vi "CODMn启动 (子VI).vi"(9 "强制切换":bool, 10 "CODMn量程切换":enum32{"H", "L", "AUTO"}(ring)=enum."AUTO", 11 "启动测量模式":T2) -> (0 "error out":T1={"status"=FALSE, "代码"=4, "source"=""} caption="错误输出" {"代码" items=["执行成功"=1, "执行失败，但不知道原因"=2, "命令请求条件错误"=3, "通讯超时"=4, "系统繁忙不能执行"=5, "系统故障"=6, "没有数据"=100]})   [LabVIEW 2016]
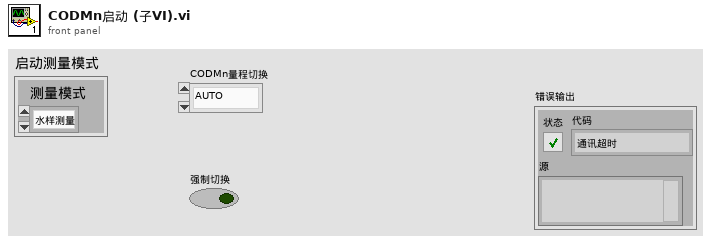
[diagram p1: front panel]
types:
  T1 = cluster{"status":bool, "代码":u16, "source":string}
  T2 = cluster{"测量模式":enum16{"水样测量", "标样核查", "零点核查", "跨度核查", "空白测试", "加标回收", "平行样", "校零", "校标"}}
  T3 = enum16{"空闲", "水样测试", "标样核查", "零点核查", "跨度核查", "空白测试", "平行样测试", "质控样", "空白校准", "标样校准", "加标回收"}
  T4 = cluster{"系统时间":timestamp, "工作状态":u16, "测量模式":enum16{"待机", "连续模式", "周期模式", "定点模式", "受控模式", "手动模式"}, "告警代码":u16, "故障代码":u16, "日志代码":u16, "软件版本":u16, "A":sgl, "B":sgl, "K":sgl, "当前滴定数":sgl, "T":sgl, "H":sgl, "id":u16, "flowid":u16, "量程":u16, "加热实时温度":sgl, "当前ORP值":sgl, "运行时间":sgl, "当前步骤剩余时间":sgl, "结束滴定数":sgl, "注射泵保温温度":sgl}
  T5 = cluster{"命令":string, "测量模式":enum16{"水样测量", "标样核查", "零点核查", "跨度核查", "空白测试", "加标回收", "平行样", "校零", "校标"}, "CODMn量程切换":enum32{"H", "L", "AUTO"}}
  T6 = enum16{"水样测量", "标样核查", "零点核查", "跨度核查", "空白测试", "加标回收", "平行样", "校零", "校标"}
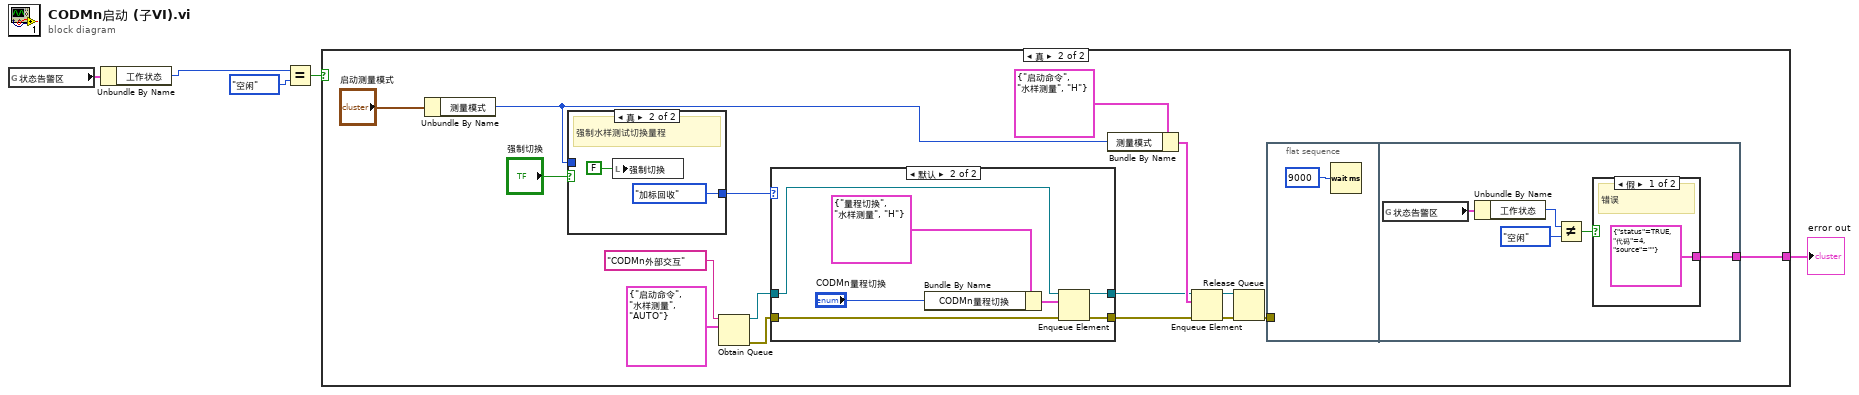
[diagram p0: block diagram]
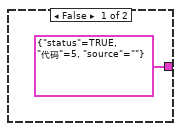
[diagram p2: hidden frame]
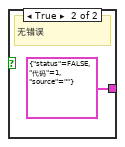
[diagram p3: hidden frame]
diagram:
  n1 = global read "VARCODMn全局变量.vi" "状态告警区"() -> (w2:T4)
  n2 = Unbundle By Name(w2) -> ("工作状态"=w1:u16)
  n3 = Equal?(x=w1, y=T3."空闲") -> (x = y?=w4:bool)
  n4 = case shown="真" w4 {
    tunnel: [T1 {"status"=TRUE, "代码"=5, "source"=""} ("error out") w7] -> w3
    frame False {
    }
    frame True {
      n5 = Unbundle By Name("启动测量模式") -> ("测量模式"=w10:T6)
      n6 = case shown="真" "强制切换" {
        tunnel: w10 -> [w31 _]
        tunnel: [w31 T6."加标回收" ("测量模式")] -> w9
        frame False {
        }
        frame True {
          # "强制水样测试切换量程"
          n7 = local write "强制切换"(FALSE ("强制切换")) -> ()
        }
      }
      n8 = Obtain Queue(name (unnamed)="CODMn外部交互" ("名称（未命名）"), element data type=T5 {"命令"="启动命令", "测量模式"=enum."水样测量", "CODMn量程切换"=enum."AUTO"} ("元素")) -> (queue out=w15:refnum<queue>, error out=w14:errorcluster)  [unwired: 3 in, 1 out]
      n9 = case shown="默认" w9 {
        tunnel: w15 -> [w35 w42]
        tunnel: w14 -> [w34 w41]
        tunnel: [w35 w40] -> w13
        tunnel: [w34 w39] -> w12
        frame "水样测量" {
        }
        frame Default {
          n10 = Bundle By Name(cluster=T5 {"命令"="量程切换", "测量模式"=enum."水样测量", "CODMn量程切换"=enum."H"} ("元素"), "CODMn量程切换"="CODMn量程切换") -> (w37:T5)
          n11 = Enqueue Element(queue=w42, element=w37, error in (no error)=w41) -> (queue out=w40:refnum<queue>, error out=w39:errorcluster)  [unwired: 1 in, 1 out]
        }
      }
      n12 = Bundle By Name(cluster=T5 {"命令"="启动命令", "测量模式"=enum."水样测量", "CODMn量程切换"=enum."H"} ("元素"), "测量模式"=w10) -> (w16:T5)
      n13 = Enqueue Element(queue=w13, element=w16, error in (no error)=w12) -> (queue out=w20:refnum<queue>, error out=w19:errorcluster)  [unwired: 1 in, 1 out]
      n14 = Release Queue(queue=w20, error in (no error)=w19) -> (error out=w8:errorcluster)  [unwired: 1 in, 2 out]
      n15 = flat-sequence {
        tunnel: w8 -> [_]
        tunnel: [w26] -> w7
        frame #0 {
          n16 = Wait (ms)(milliseconds to wait=u32 9000 ("等待时间（毫秒）")) -> ()  [unwired: 1 out]
        }
        frame #1 {
          n17 = global read "VARCODMn全局变量.vi" "状态告警区"() -> (w25:T4)
          n18 = Unbundle By Name(w25) -> ("工作状态"=w24:u16)
          n19 = Not Equal?(x=w24, y=T3."空闲") -> (x != y?=w27:bool)
          n20 = case shown="假" w27 {
            tunnel: [T1 {"status"=TRUE, "代码"=4, "source"=""} ("error out") T1 {"status"=FALSE, "代码"=1, "source"=""} ("error out")] -> w26
            frame False {
              # "错误"
            }
            frame True {
              # "无错误"
            }
          }
        }
      }
    }
  }
  "error out" <- w3
